vi "CheckSwallow.vi"(8 "error in (no error)":errorcluster, 10 "Snake.lvclass":refnum<class "Snake.lvclass">, 11 "Feeder in":refnum<class "Feeder.lvclass">) -> (0 "error out":errorcluster, 2 "Swallowed?":bool, 3 "Feeder out":refnum<class "Feeder.lvclass">)   [LabVIEW 2018, in "Feeder.lvclass"]
uses:
  Feeder.lvclass
  Snake/Snake.lvclass
  Feeder.lvclass/Feeder.ctl
panel:
  # "Connector Pane"
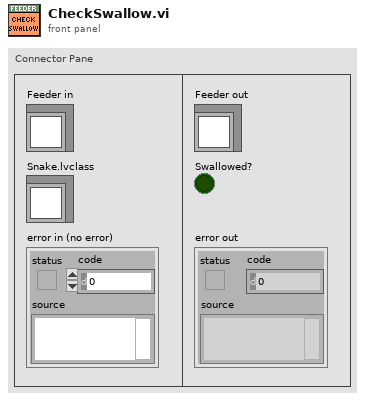
[diagram p1: front panel]
types:
  T1 = typedef "XYposition.ctl" = cluster{"Col.LocX":i32, "Row.LocY":i32}
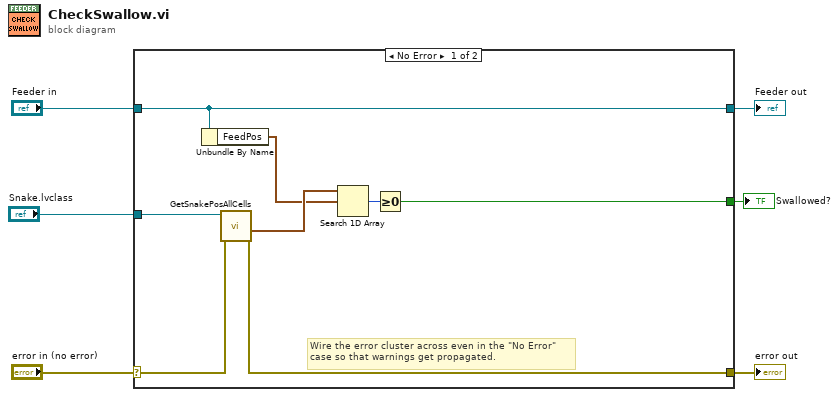
[diagram p0: block diagram]
diagram:
  n1 = case shown="No Error" "error in (no error)" {
    selector: "error in (no error)" -> [w13 w16]
    tunnel: [w12 w16] -> w5
    tunnel: [w11 w15] -> w3
    tunnel: "Feeder in" -> [w11 w15]
    tunnel: "Snake.lvclass" -> [w14 _]
    tunnel: [w7 _] -> w1
    frame No Error {
      # "Wire the error cluster across even in the \"No Error\"\ncase so that warnings get propagated."
      n2 = Unbundle By Name(w11) -> ("FeedPos"=w9:T1)
      n3 = call "GetSnakePosAllCells.vi"("error in (no error)"=w13, "Snake in"=w14) -> ("error out"=w12:errorcluster, "CellPositions"=w10:T1[])  [unwired: 6 in, 2 out]
      n4 = Search 1D Array(1D array=w10, element=w9) -> (index of element=w8:i32)  [unwired: 1 in]
      n5 = Greater Or Equal To 0?(x=w8) -> (x >= 0?=w7:bool)
    }
    frame Error {
    }
  }
  "error out" <- w5
  "Feeder out" <- w3
  "Swallowed?" <- w1
